vi "PeaksInPlotV0.54.vi"(0 "Format String":string, 1 "Unit String":string, 2 "X-Axis Array":dbl[][](array[numeric]) format="%.2f", 3 "Data Array":dbl[][](array[numeric]) format="%.2f", 4 "Cursor Plot":u32) -> (5 "Peaks: X":dbl[](array[numeric]) format="%.3f", 6 "Peak Position Strings []":string[](array[string]), 7 "Peaks: Y":dbl[](array[numeric]) format="%.3e")   [LabVIEW 2019]
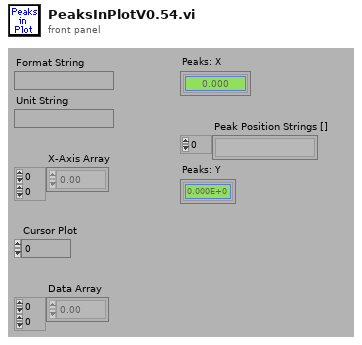
[diagram p1: front panel]
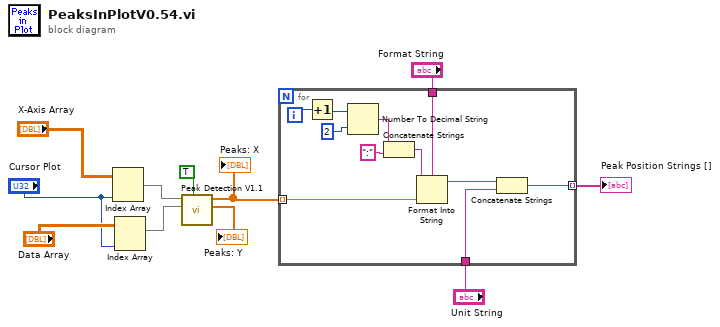
[diagram p0: block diagram]
diagram:
  n1 = Index Array(array="X-Axis Array", index (col)="Cursor Plot") -> (element=w4:dbl[])  [unwired: 1 in]
  n2 = Index Array(array="Data Array", index (col)="Cursor Plot") -> (element=w5:dbl[])  [unwired: 1 in]
  n3 = call "Peak Detection V1.1.vi"("View Result?"=TRUE, "Input y data"=w5, "Input x data"=w4) -> ("Peak Amplitudes"=→"Peaks: Y":dbl[], "Peak Locations"=w8:dbl[])  [unwired: 2 in, 5 out]
  "Peaks: X" <- w8
  n4 = for {
    tunnel: w8 -> [w22] mode=indexing
    tunnel: "Format String" -> [w17]
    tunnel: [w14] -> w9 mode=indexing
    tunnel: "Unit String" -> [w15]
    i -> [w12]
    n5 = Increment(x=w12) -> (x+1=w13:i32)
    n6 = Number To Decimal String(number=w13, width (-)=i16 2) -> (decimal integer string=w20:string)
    n7 = Concatenate Strings(w20, ":") -> (w18:string)
    n8 = Format Into String(format string=w17, initial string=w18, w22) -> (resulting string=w16:string)  [unwired: 1 in, 1 out]
    n9 = Concatenate Strings(w16, w15) -> (w14:string)
  }
  "Peak Position Strings []" <- w9
